vi "Psi.vi"(4 "dt [s]":dbl, 5 "error in (no error)":errorcluster, 6 "model description":T8={"model"="sin(x+a0)", "Parameters"=["a0"], "x"="x"}, 7 "Data before TCT":T1, 8 "Params in":T2={"TaskIDs"={"DAQ tasks"={"Px taskID"=0, "Py taskID"=0, "Pz taskID"=0, "AOM taskID"=0, "Clock taskID"=0, "AI taskID"=0}, "DVEHandle"=refnum}, "Manual Control"={"Rotation Control"={"Phase"=0.0, "A amp (0-120)"=75.0, "B amp (0-120)"=53.3, "mean freq  [MHz]\ndefault 39.99"=40.0, "freq difference [Hz]"=2.0, "Enable A"=TRUE, "Enable B"=TRUE}, "X piezo\n [nm]"=0.0, "Y peizo\n [nm]"=0.0, "trap height\n [nm]"=5.012658227848101, "AOM0 \nPower"=0.2}, "Piezo Calibr"={"Px2Vx(AO)"=nan, "Py2Vy(AO)"=nan, "Pz2Vz(AO)"=nan, "Min Px"=nan, "Min Py"=nan, "Min Pz"=nan, "Max Px"=nan, "Max Py"=nan, "Max Pz"=nan, "Vx0 (V)"=nan, "Vy0 (V)"=nan, "Vz0 (V)"=nan}, "Instrument Calibr"={"Angular compensation coeffs"=[], "TetherCenter"={"TrapX_AO 0 [nm]"=nan, "TrapY_AO 0 [nm]"=nan, "TrapZ_AO 0 [nm]"=nan}, "XYZsignal baseline"={"Xsignal0"=nan, "Ysignal0"=nan, "Zsignal0"=nan, "Zsig slope"=nan, "Z bead0"=nan}, "S and P to Vs0"={"Vs0/P"=1.0, "Vs0/S"=1.0}, "Psi"=0.0, "ePS:eRL drift correlation"={"Interc P"=nan, "Slope P"=nan, "Interc S"=nan, "Slope S"=nan}, "Current piezo volt AO"={"Vpx_AO [V]"=nan, "Vpy_AO [V]"=nan, "Vpz_AO [V]"=nan}}, "Cylinder Calibr"={"ZStiff"=nan, "Zsens"=nan, "AngStiff"=nan, "XStiff"=nan, "Xsens"=nan, "MaxEllip"=nan, "YStiff"=nan, "Ysens"=nan, "FocalShift"=nan, "Sfz"=nan, "1/Sz"=nan, "Stau"=nan, "Sfx"=nan, "1/Sx"=nan, "1/Sang"=nan, "Sfy"=nan, "1/Sy"=nan, "1/focal"=nan, "ZsignalHeightDependence (1/nm)"=0.0}, "DAQParams"={"Buffer size"=nan, "Scanning rate"=nan, "Average"=nan, "Sampling rate"=nan, "set dt"=nan}, "DAQ channel offsets"={"A0 [V]"=0.0, "D0 [V]"=0.0, "P0  [V]"=0.0, "S0 [V]"=0.0, "L0 [V]"=0.0, "R0 [V]"=0.0, "Vpx0 [V]"=0.0, "Vpy0 [V]"=0.0, "Vpz0 [V]"=0.0, "Vsum0 [V]"=0.0, "Vpx_AO0 [V]"=0.0, "Vpy_AO0 [V]"=0.0, "Vpz_AO0 [V]"=0.0}, "Z bead polynomial coeffs"=[nan, nan, nan, nan], "Skip button ref"=refnum, "z bead lookup table"={"z signal"=[], "z bead"=[]}, "SP->power Matrix"=[], "Ms2p"=[], "Mp2s"=[], "Polynomial coeff V_px,y,z 2 position (nm)"=[]} {"Cylinder Calibr"."ZsignalHeightDependence (1/nm)" format="%.4e"; "Instrument Calibr"."Psi" format="%#_2f"; "Manual Control"."Y peizo\n [nm]" step=100.0 scale=0.0..30000.0; "Manual Control"."AOM0 \nPower" scale=0.0..1.0; "Manual Control"."X piezo\n [nm]" step=100.0 scale=0.0..30000.0; "Manual Control"."Rotation Control"."mean freq  [MHz]\ndefault 39.99" min=0.0 step=0.01; "Manual Control"."Rotation Control"."B amp (0-120)" min=0.0 max=120.0 step=0.1 format="%.1f"; "Manual Control"."Rotation Control"."A amp (0-120)" min=0.0 max=120.0 step=0.1 format="%.1f"; "Manual Control"."Rotation Control"."Phase" scale=0.0..360.0; "Manual Control"."trap height\n [nm]" scale=1000.0..7500.0; "TaskIDs"."DAQ tasks"."Px taskID" format="%x"; "TaskIDs"."DAQ tasks"."Py taskID" format="%x"; "TaskIDs"."DAQ tasks"."Pz taskID" format="%x"; "TaskIDs"."DAQ tasks"."AOM taskID" format="%x"; "TaskIDs"."DAQ tasks"."Clock taskID" format="%x"; "TaskIDs"."DAQ tasks"."AI taskID" format="%x"}) -> (0 "error out":errorcluster, 1 "Psi":dbl, 3 "Params out":T2={"TaskIDs"={"DAQ tasks"={"Px taskID"=0, "Py taskID"=0, "Pz taskID"=0, "AOM taskID"=0, "Clock taskID"=0, "AI taskID"=0}, "DVEHandle"=refnum}, "Manual Control"={"Rotation Control"={"Phase"=0.0, "A amp (0-120)"=75.0, "B amp (0-120)"=53.3, "mean freq  [MHz]\ndefault 39.99"=40.0, "freq difference [Hz]"=2.0, "Enable A"=TRUE, "Enable B"=TRUE}, "X piezo\n [nm]"=0.0, "Y peizo\n [nm]"=0.0, "trap height\n [nm]"=5.012658227848101, "AOM0 \nPower"=0.2}, "Piezo Calibr"={"Px2Vx(AO)"=nan, "Py2Vy(AO)"=nan, "Pz2Vz(AO)"=nan, "Min Px"=nan, "Min Py"=nan, "Min Pz"=nan, "Max Px"=nan, "Max Py"=nan, "Max Pz"=nan, "Vx0 (V)"=nan, "Vy0 (V)"=nan, "Vz0 (V)"=nan}, "Instrument Calibr"={"Angular compensation coeffs"=[], "TetherCenter"={"TrapX_AO 0 [nm]"=nan, "TrapY_AO 0 [nm]"=nan, "TrapZ_AO 0 [nm]"=nan}, "XYZsignal baseline"={"Xsignal0"=nan, "Ysignal0"=nan, "Zsignal0"=nan, "Zsig slope"=nan, "Z bead0"=nan}, "S and P to Vs0"={"Vs0/P"=1.0, "Vs0/S"=1.0}, "Psi"=0.0, "ePS:eRL drift correlation"={"Interc P"=nan, "Slope P"=nan, "Interc S"=nan, "Slope S"=nan}, "Current piezo volt AO"={"Vpx_AO [V]"=nan, "Vpy_AO [V]"=nan, "Vpz_AO [V]"=nan}}, "Cylinder Calibr"={"ZStiff"=nan, "Zsens"=nan, "AngStiff"=nan, "XStiff"=nan, "Xsens"=nan, "MaxEllip"=nan, "YStiff"=nan, "Ysens"=nan, "FocalShift"=nan, "Sfz"=nan, "1/Sz"=nan, "Stau"=nan, "Sfx"=nan, "1/Sx"=nan, "1/Sang"=nan, "Sfy"=nan, "1/Sy"=nan, "1/focal"=nan, "ZsignalHeightDependence (1/nm)"=0.0}, "DAQParams"={"Buffer size"=nan, "Scanning rate"=nan, "Average"=nan, "Sampling rate"=nan, "set dt"=nan}, "DAQ channel offsets"={"A0 [V]"=0.0, "D0 [V]"=0.0, "P0  [V]"=0.0, "S0 [V]"=0.0, "L0 [V]"=0.0, "R0 [V]"=0.0, "Vpx0 [V]"=0.0, "Vpy0 [V]"=0.0, "Vpz0 [V]"=0.0, "Vsum0 [V]"=0.0, "Vpx_AO0 [V]"=0.0, "Vpy_AO0 [V]"=0.0, "Vpz_AO0 [V]"=0.0}, "Z bead polynomial coeffs"=[nan, nan, nan, nan], "Skip button ref"=refnum, "z bead lookup table"={"z signal"=[], "z bead"=[]}, "SP->power Matrix"=[], "Ms2p"=[], "Mp2s"=[], "Polynomial coeff V_px,y,z 2 position (nm)"=[]} {"Cylinder Calibr"."ZsignalHeightDependence (1/nm)" format="%.4e"; "Instrument Calibr"."Psi" format="%#_2f"; "Manual Control"."Y peizo\n [nm]" step=100.0 scale=0.0..30000.0; "Manual Control"."AOM0 \nPower" scale=0.0..1.0; "Manual Control"."X piezo\n [nm]" step=100.0 scale=0.0..30000.0; "Manual Control"."Rotation Control"."mean freq  [MHz]\ndefault 39.99" min=0.0 step=0.01; "Manual Control"."Rotation Control"."B amp (0-120)" min=0.0 max=120.0 step=0.1 format="%.1f"; "Manual Control"."Rotation Control"."A amp (0-120)" min=0.0 max=120.0 step=0.1 format="%.1f"; "Manual Control"."Rotation Control"."Phase" scale=0.0..360.0; "Manual Control"."trap height\n [nm]" scale=1000.0..7500.0; "TaskIDs"."DAQ tasks"."Px taskID" format="%x"; "TaskIDs"."DAQ tasks"."Py taskID" format="%x"; "TaskIDs"."DAQ tasks"."Pz taskID" format="%x"; "TaskIDs"."DAQ tasks"."AOM taskID" format="%x"; "TaskIDs"."DAQ tasks"."Clock taskID" format="%x"; "TaskIDs"."DAQ tasks"."AI taskID" format="%x"})   [LabVIEW 2020, in "SignalConverson.lvlib"]
uses:
  SignalConverson.lvlib
  Initialization/Param.ctl
  Initialization/ManualCtrl.ctl
  Initialization/DVESetting.ctl
  Initialization/CylinderCalibrNew.ctl
  DAQChannelOffsets.ctl
  <vilib>/Analysis/Matrix/Datatypes/RealMatrix.ctl
  Data Before Angle Compensation.ctl
  <vilib>/gmath/NumericalOptimization/Nonlinear Curve Fit LM formula string.vi
  <vilib>/gmath/NI_Gmath.lvlib
  Initialization/Initialization.lvlib
  <vilib>/Analysis/Matrix/NI_Matrix.lvlib
panel:
  in  "Tab Control":enum32{"data", "plot of fitting"}(tab)
  out "XY Graph":cluster{dbl[], "best fit parameters":dbl[]}[](graph)
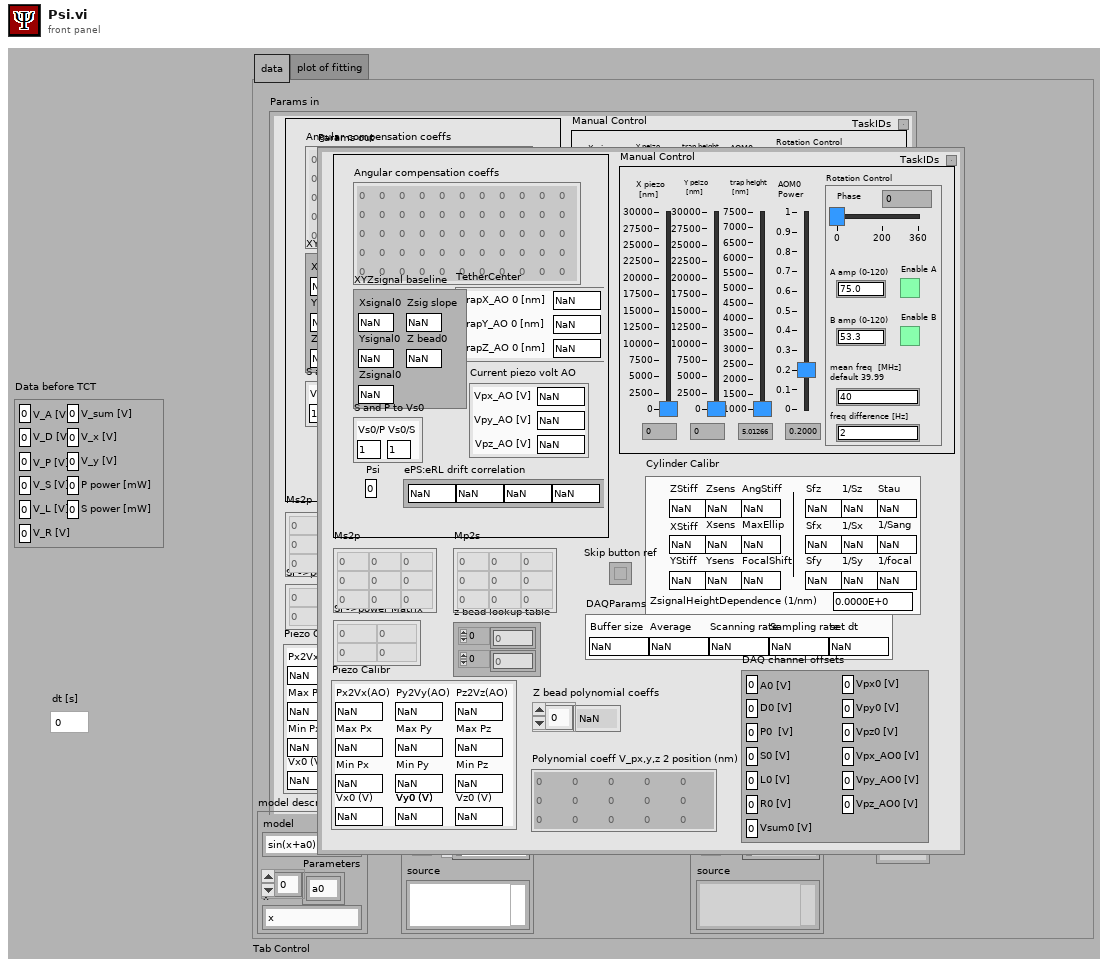
[diagram p1: front panel]
types:
  T1 = typedef "SignalConverson.lvlib/Data Before Angle Compensation.ctl" = cluster{"V_A [V]":dbl, "V_D [V]":dbl, "V_P [V]":dbl, "V_S [V]":dbl, "V_L [V]":dbl, "V_R [V]":dbl, "V_sum [V]":dbl, "V_x [V]":dbl, "V_y [V]":dbl, "P power [mW]":dbl, "S power [mW]":dbl}
  T2 = typedef "Initialization.lvlib/Param.ctl" = cluster{"TaskIDs":cluster{"DAQ tasks":cluster{"Px taskID":u32, "Py taskID":u32, "Pz taskID":u32, "AOM taskID":u32, "Clock taskID":u32, "AI taskID":u32}, "DVEHandle":refnum<file>}, "Manual Control":T3, "Piezo Calibr":cluster{"Px2Vx(AO)":dbl, "Py2Vy(AO)":dbl, "Pz2Vz(AO)":dbl, "Min Px":dbl, "Min Py":dbl, "Min Pz":dbl, "Max Px":dbl, "Max Py":dbl, "Max Pz":dbl, "Vx0 (V)":dbl, "Vy0 (V)":dbl, "Vz0 (V)":dbl}, "Instrument Calibr":cluster{"Angular compensation coeffs":dbl[][], "TetherCenter":cluster{"TrapX_AO 0 [nm]":dbl, "TrapY_AO 0 [nm]":dbl, "TrapZ_AO 0 [nm]":dbl}, "XYZsignal baseline":cluster{"Xsignal0":dbl, "Ysignal0":dbl, "Zsignal0":dbl, "Zsig slope":dbl, "Z bead0":dbl}, "S and P to Vs0":cluster{"Vs0/P":dbl, "Vs0/S":dbl}, "Psi":dbl, "ePS:eRL drift correlation":cluster{"Interc P":dbl, "Slope P":dbl, "Interc S":dbl, "Slope S":dbl}, "Current piezo volt AO":cluster{"Vpx_AO [V]":dbl, "Vpy_AO [V]":dbl, "Vpz_AO [V]":dbl}}, "Cylinder Calibr":T5, "DAQParams":cluster{"Buffer size":dbl, "Scanning rate":dbl, "Average":dbl, "Sampling rate":dbl, "set dt":dbl}, "DAQ channel offsets":T6, "Z bead polynomial coeffs":dbl[], "Skip button ref":refnum<vi>, "z bead lookup table":cluster{"z signal":dbl[], "z bead":dbl[]}, "SP->power Matrix":T7, "Ms2p":T7, "Mp2s":T7, "Polynomial coeff V_px,y,z 2 position (nm)":dbl[][]}
  T3 = typedef "Initialization.lvlib/ManualCtrl.ctl" = cluster{"Rotation Control":T4, "X piezo\n [nm]":dbl, "Y peizo\n [nm]":dbl, "trap height\n [nm]":dbl, "AOM0 \nPower":dbl}
  T4 = typedef "Initialization.lvlib/DVESetting.ctl" = cluster{"Phase":dbl, "A amp (0-120)":dbl, "B amp (0-120)":dbl, "mean freq  [MHz]\ndefault 39.99":dbl, "freq difference [Hz]":dbl, "Enable A":bool, "Enable B":bool}
  T5 = typedef "Initialization.lvlib/CylinderCalibrNew.ctl" = cluster{"ZStiff":dbl, "Zsens":dbl, "AngStiff":dbl, "XStiff":dbl, "Xsens":dbl, "MaxEllip":dbl, "YStiff":dbl, "Ysens":dbl, "FocalShift":dbl, "Sfz":dbl, "1/Sz":dbl, "Stau":dbl, "Sfx":dbl, "1/Sx":dbl, "1/Sang":dbl, "Sfy":dbl, "1/Sy":dbl, "1/focal":dbl, "ZsignalHeightDependence (1/nm)":dbl}
  T6 = typedef "SignalConverson.lvlib/DAQChannelOffsets.ctl" = cluster{"A0 [V]":dbl, "D0 [V]":dbl, "P0  [V]":dbl, "S0 [V]":dbl, "L0 [V]":dbl, "R0 [V]":dbl, "Vpx0 [V]":dbl, "Vpy0 [V]":dbl, "Vpz0 [V]":dbl, "Vsum0 [V]":dbl, "Vpx_AO0 [V]":dbl, "Vpy_AO0 [V]":dbl, "Vpz_AO0 [V]":dbl}
  T7 = typedef "NI_Matrix.lvlib/RealMatrix.ctl" = dbl[][]
  T8 = cluster{"model":string, "Parameters":string[], "x":string}
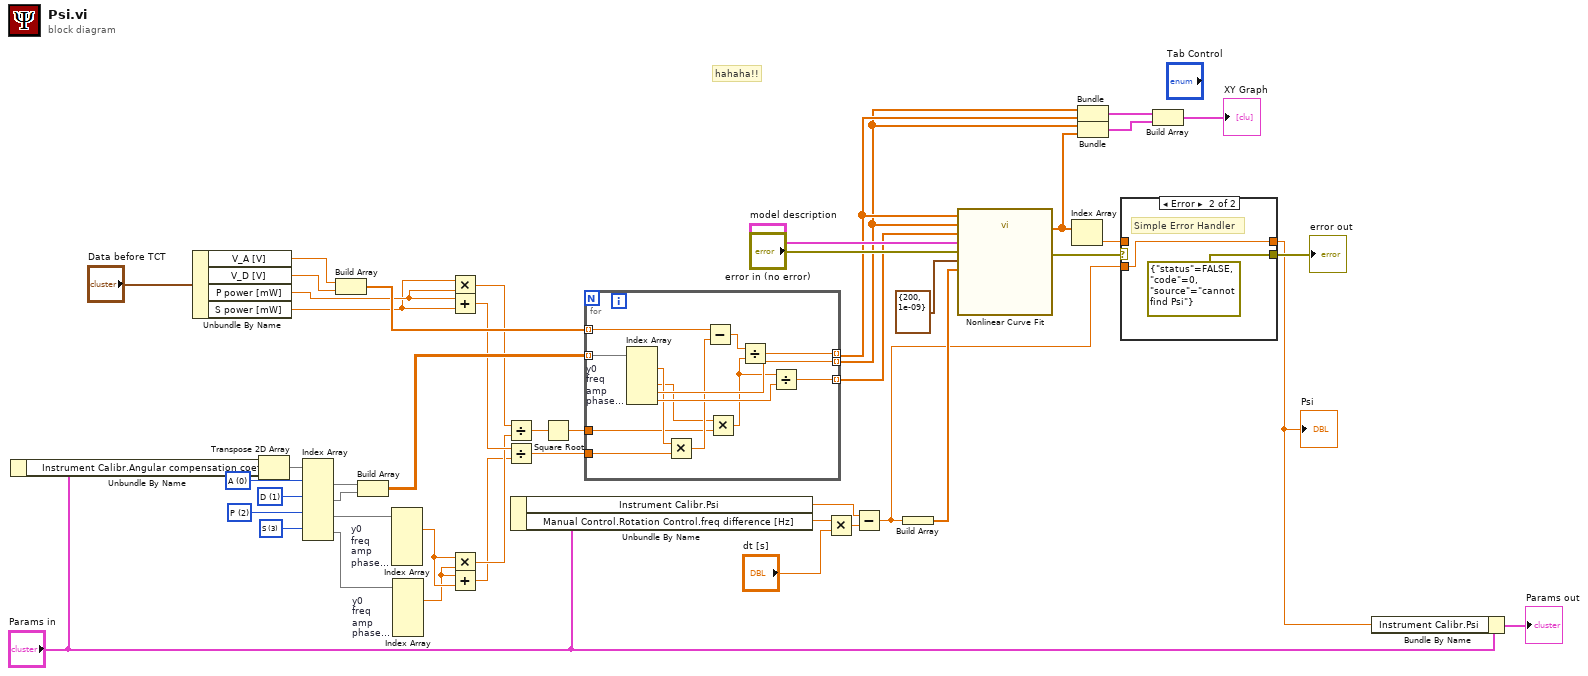
[diagram p0: block diagram]
diagram:
  w36 = 3 items=["A", "D", "P", "S", "L", "R", "Vsum", "Vx", "Vy", "Piezo U", "Piezo V", "Piezo Z"] ("Channel 3")
  w37 = 2 items=["A", "D", "P", "S", "L", "R", "Vsum", "Vx", "Vy", "Piezo U", "Piezo V", "Piezo Z"] ("Channel 3")
  w38 = 1 items=["A", "D", "P", "S", "L", "R", "Vsum", "Vx", "Vy", "Piezo U", "Piezo V", "Piezo Z"] ("Channel 3")
  w39 = 0 items=["A", "D", "P", "S", "L", "R", "Vsum", "Vx", "Vy", "Piezo U", "Piezo V", "Piezo Z"] ("Channel 3")
  # "hahaha!!"
  n1 = Unbundle By Name("Params in") -> ("Instrument Calibr.Angular compensation coeffs"=w40:dbl[][])
  n2 = Unbundle By Name("Data before TCT") -> ("V_A [V]"=w4:dbl, "V_D [V]"=w3:dbl, "P power [mW]"=w2:dbl, "S power [mW]"=w1:dbl)
  n3 = Transpose 2D Array(2D array=w40) -> (transposed array=w33:dbl[][])
  n4 = Index Array(array=w33, index (row) #1=w39, index (row) #2=w38, index (row) #3=w37, index (row) #4=w36) -> (element #1=w35:dbl[], element #2=w34:dbl[], element #3=w30:dbl[], element #4=w29:dbl[])  [unwired: 4 in]
  n5 = Build Array(w4, w3) -> (w31:dbl[])
  n6 = Build Array(w35, w34) -> (w32:dbl[][])
  n7 = Index Array "y0\nfreq\namp\nphase\nresidue"(array=w30) -> (element #1=w28:dbl)  [unwired: 5 in, 4 out]
  n8 = Index Array "y0\nfreq\namp\nphase\nresidue"(array=w29) -> (element #1=w27:dbl)  [unwired: 5 in, 4 out]
  n9 = Multiply(x=w1, y=w2) -> (x*y=w26:dbl)
  n10 = Add(x=w2, y=w1) -> (x+y=w25:dbl)
  n11 = Multiply(x=w28, y=w27) -> (x*y=w24:dbl)
  n12 = Add(x=w27, y=w28) -> (x+y=w23:dbl)
  n13 = Divide(x=w26, y=w24) -> (x/y=w22:dbl)
  n14 = Divide(x=w25, y=w23) -> (x/y=w21:dbl)
  n15 = Unbundle By Name("Params in") -> ("Instrument Calibr.Psi"=w8:dbl, "Manual Control.Rotation Control.freq difference [Hz]"=w10:dbl)
  n16 = Square Root(x=w22) -> (sqrt(x)=w20:dbl)
  n17 = for {
    tunnel: w32 -> [w61] mode=indexing
    tunnel: w31 -> [w59] mode=indexing
    tunnel: [w58] -> w16 mode=indexing
    tunnel: [w57] -> w14 mode=indexing
    tunnel: [w55] -> w45 mode=indexing
    tunnel: w21 -> [w54]
    tunnel: w20 -> [w51]
    n18 = Index Array "y0\nfreq\namp\nphase\nresidue"(array=w61) -> (element #1=w53:dbl, element #3=w50:dbl, element #4=w57:dbl, element #5=w56:dbl)  [unwired: 5 in, 1 out]
    n19 = Multiply(x=w53, y=w54) -> (x*y=w52:dbl)
    n20 = Subtract(x=w59, y=w52) -> (x-y=w60:dbl)
    n21 = Multiply(x=w50, y=w51) -> (x*y=w49:dbl)
    n22 = Divide(x=w60, y=w49) -> (x/y=w58:dbl)
    n23 = Divide(x=w49, y=w56) -> (x/y=w55:dbl)
  }
  n24 = Multiply(x=w10, y="dt [s]") -> (x*y=w9:dbl)
  n25 = Subtract(x=w8, y=w9) -> (x-y=w7:dbl)
  n26 = Build Array(w7) -> (w44:dbl[])
  n27 = call-poly <vilib>:"Nonlinear Curve Fit.vi"("Y"=w16, "initial parameters"=w44, "X"=w14, "Weight"=w45, "model description"="model description", "error in (no error)"="error in (no error)", "termination"=cluster{"max iteration":i32, "tolerance":dbl} {"max iteration"=200, "tolerance"=1e-09}) -> ("best fit parameters"=w15:dbl[], "error out"=w43:errorcluster)  [unwired: 4 in, 3 out]
  n28 = Index Array(array=w15) -> (element=w42:dbl)  [unwired: 1 in]
  n29 = Bundle(w14, w16) -> (w13:cluster{dbl[], dbl[]})  [unwired: 1 in]
  n30 = Bundle(w14, "best fit parameters"=w15) -> (w12:cluster{dbl[], "best fit parameters":dbl[]})  [unwired: 1 in]
  n31 = case shown="Error" w43 {
    selector: w43 -> [w62 _]
    tunnel: w42 -> [w63 _]
    tunnel: w7 -> [_ w65]
    tunnel: [w63 w65] -> w17
    tunnel: [w62 errorcluster {"status"=FALSE, "code"=0, "source"="cannot find Psi"} ("error in (no error) 2")] -> w41
    frame No Error {
    }
    frame Error {
      # "Simple Error Handler"
    }
  }
  "error out" <- w41
  "Psi" <- w17
  n32 = Build Array(w13, w12) -> (→"XY Graph":cluster{dbl[], "best fit parameters":dbl[]}[])
  n33 = Bundle By Name(cluster="Params in", "Instrument Calibr.Psi"=w17) -> (→"Params out":T2)
